vi "L2R_v2.vi"() -> ()   [LabVIEW 2022 SP3]
uses:
  <vilib>/regexp/Match Regular Expression.xnode
panel:
  in  "SET_term_z_offs":dbl=20.0 caption="terminal z \noffset:"
  in  "SET_term_moc":u16(ring) caption="terminal\nmovement:" items=["none", "inside", "-X", "-Y", "Z only"]
  in  "SET_x_offs":dbl caption="X offset:"
  in  "SET_y_offs":dbl caption="Y offset:"
  out "OUT_choice":bool
  out "OUT_file_num":i32 caption="split files created"
  out "CONV_splitting":bool caption="FILE SPLITTING"
  out "OUT_comm_lines":i32 caption="command lines found"
  in  "SET_max_lines":i32=2000 caption="max. file lines"
  in  "SET_tool_angl":bool caption="tool \nangulation:"
  out "FILE_name_old":string caption="old\nfilename:"
  in  "FILE_name_new":string caption="new \nfilename:"
  in  "SET_zone":i32=10 caption="zone:"
  in  "SET_tool":string="tool0" caption="tool:"
  in  "SET_movtype":u16(ring) caption="movement \ntype:" items=["LINEAR", "JOINT"]
  out "ERR_write_file":errorcluster
  out "OUT_rapid":string caption="RAPID string"
  out "CONV_running":bool caption="CONVERSION RUNNING"
  out "ERR_read_file":errorcluster caption="read file error"
  in  "FILE_path":path caption="file path:\n(dialog)"
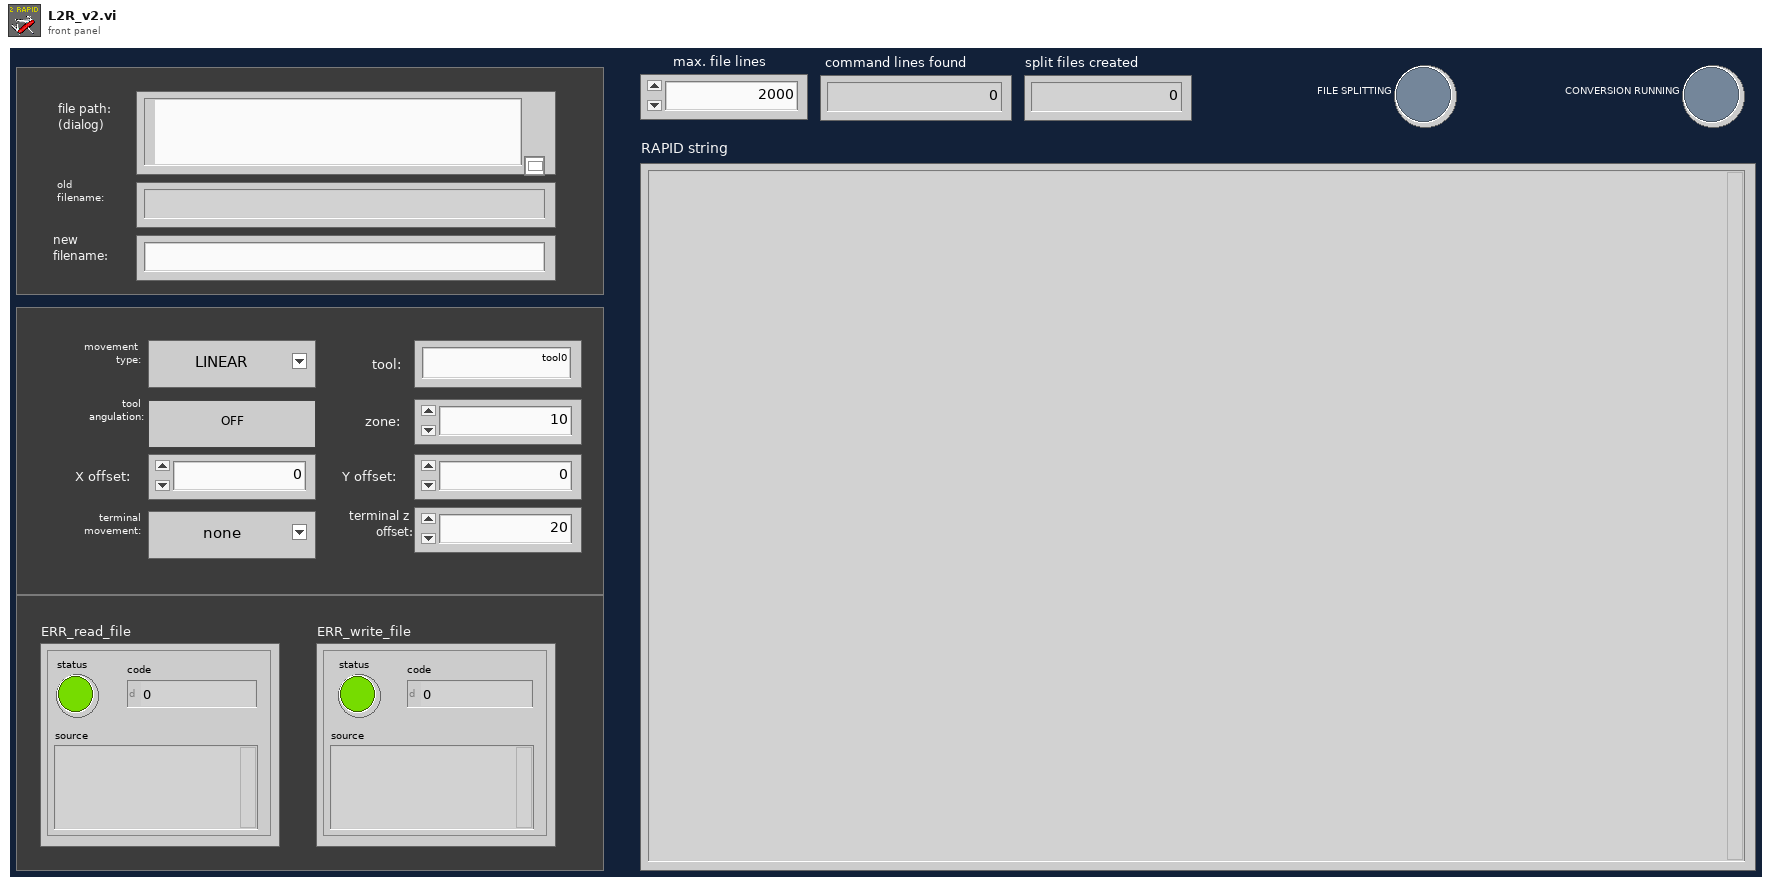
[diagram p1: front panel]
types:
  T1 = enum16{"open", "replace", "create", "open or create", "replace or create", "replace or create with confirmation"}
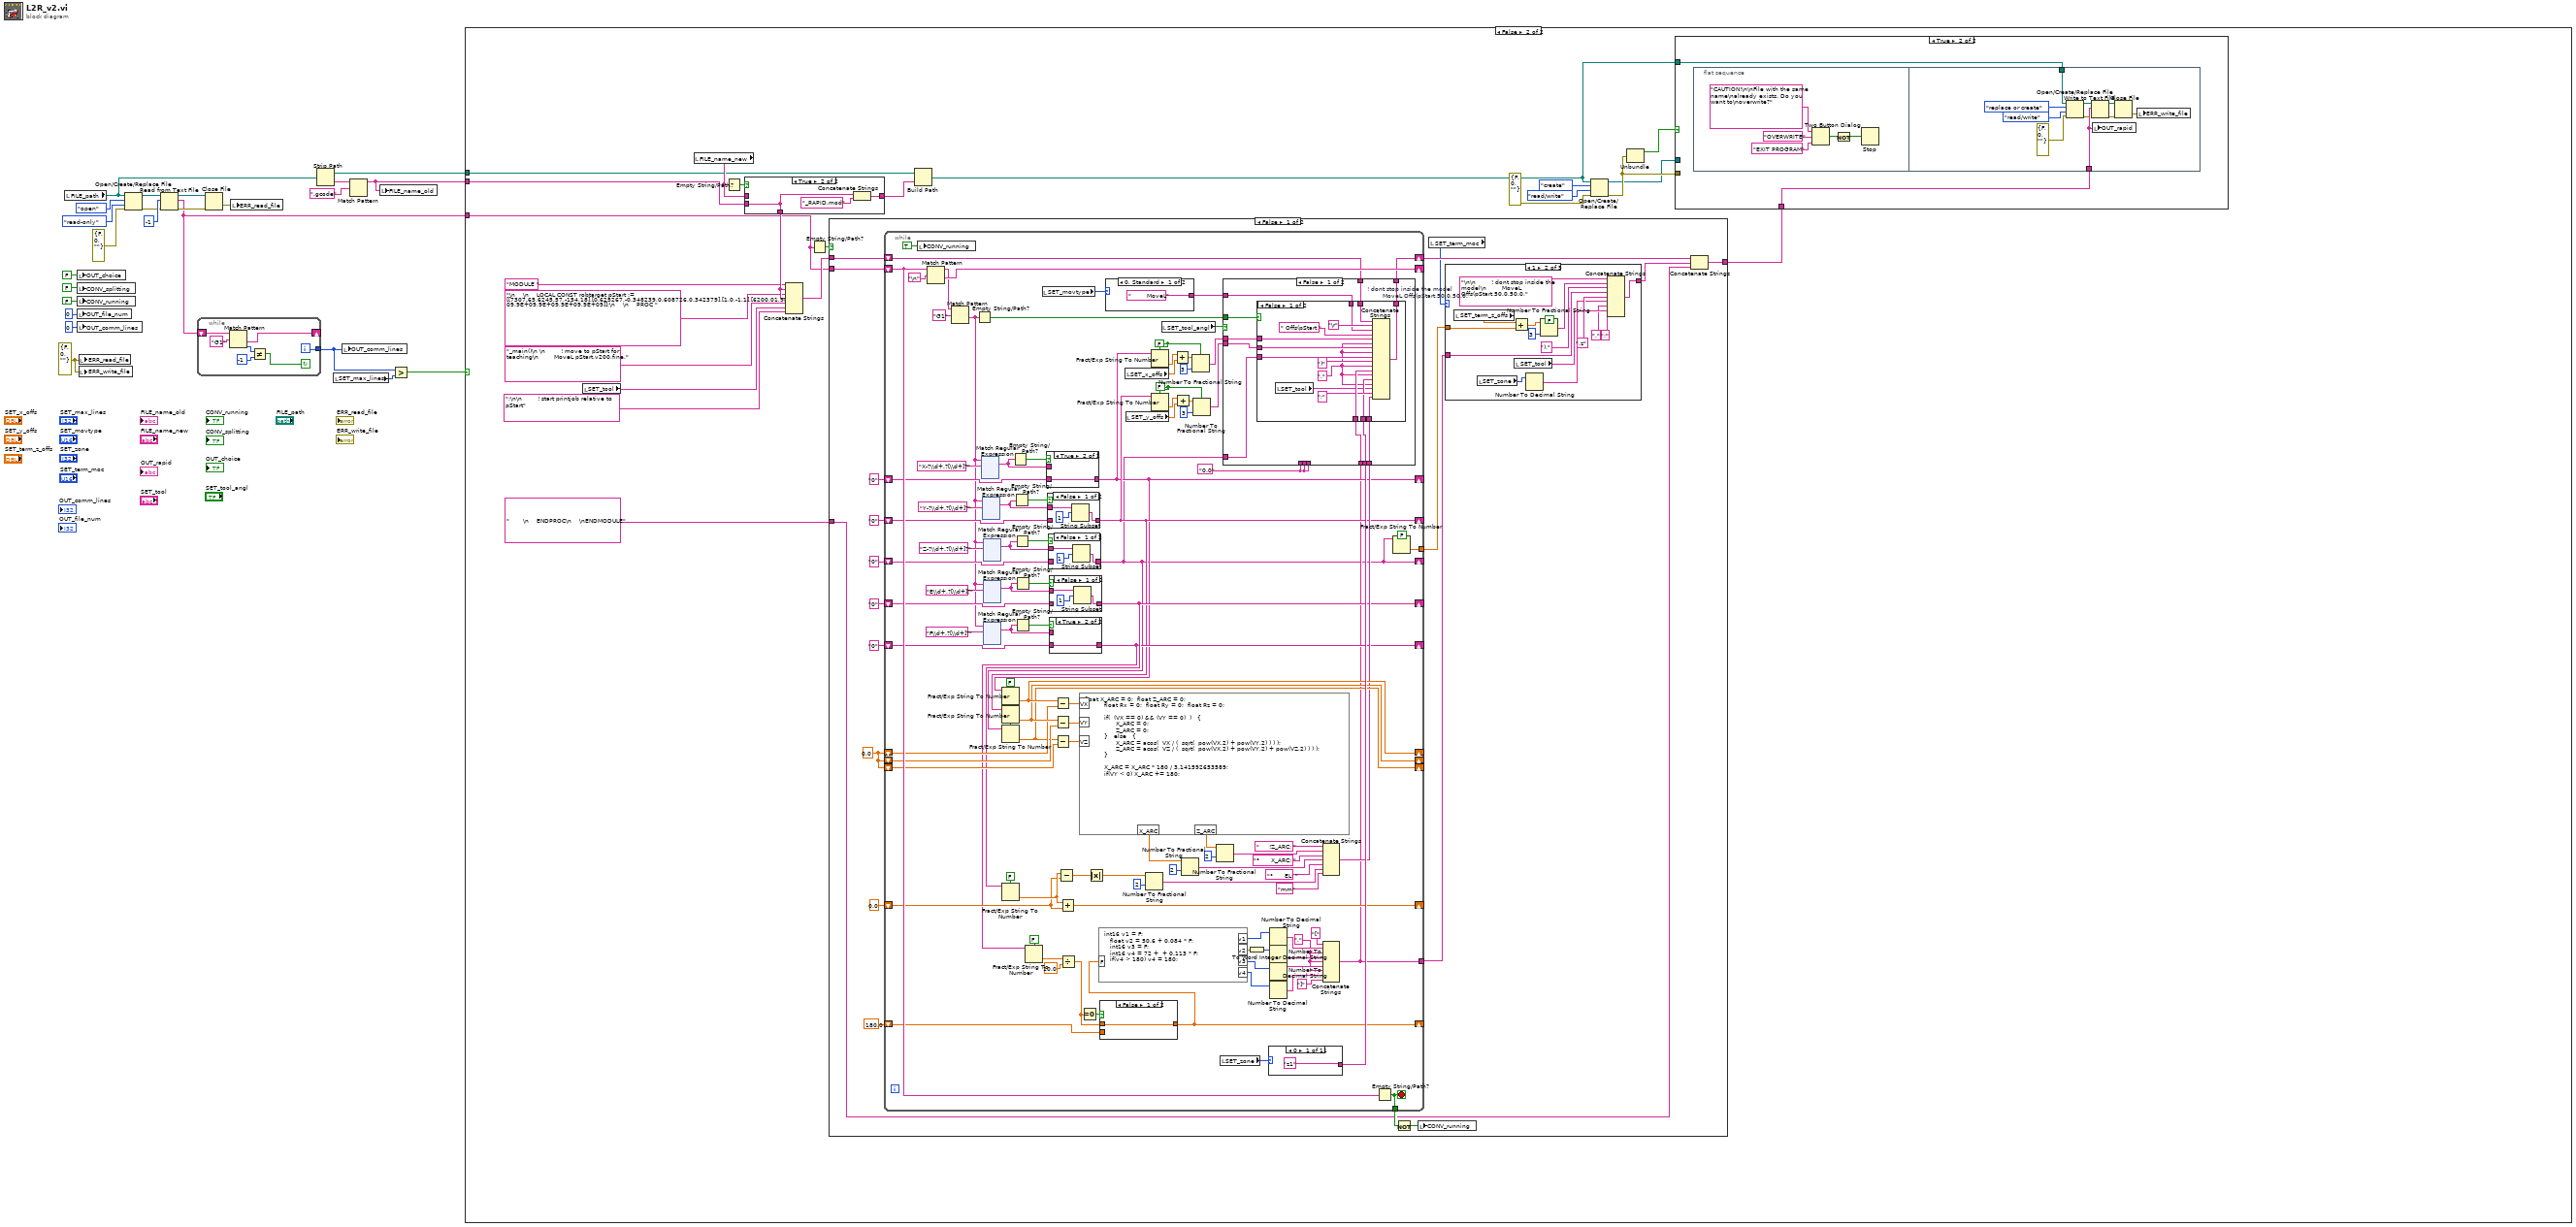
[diagram p0: block diagram]
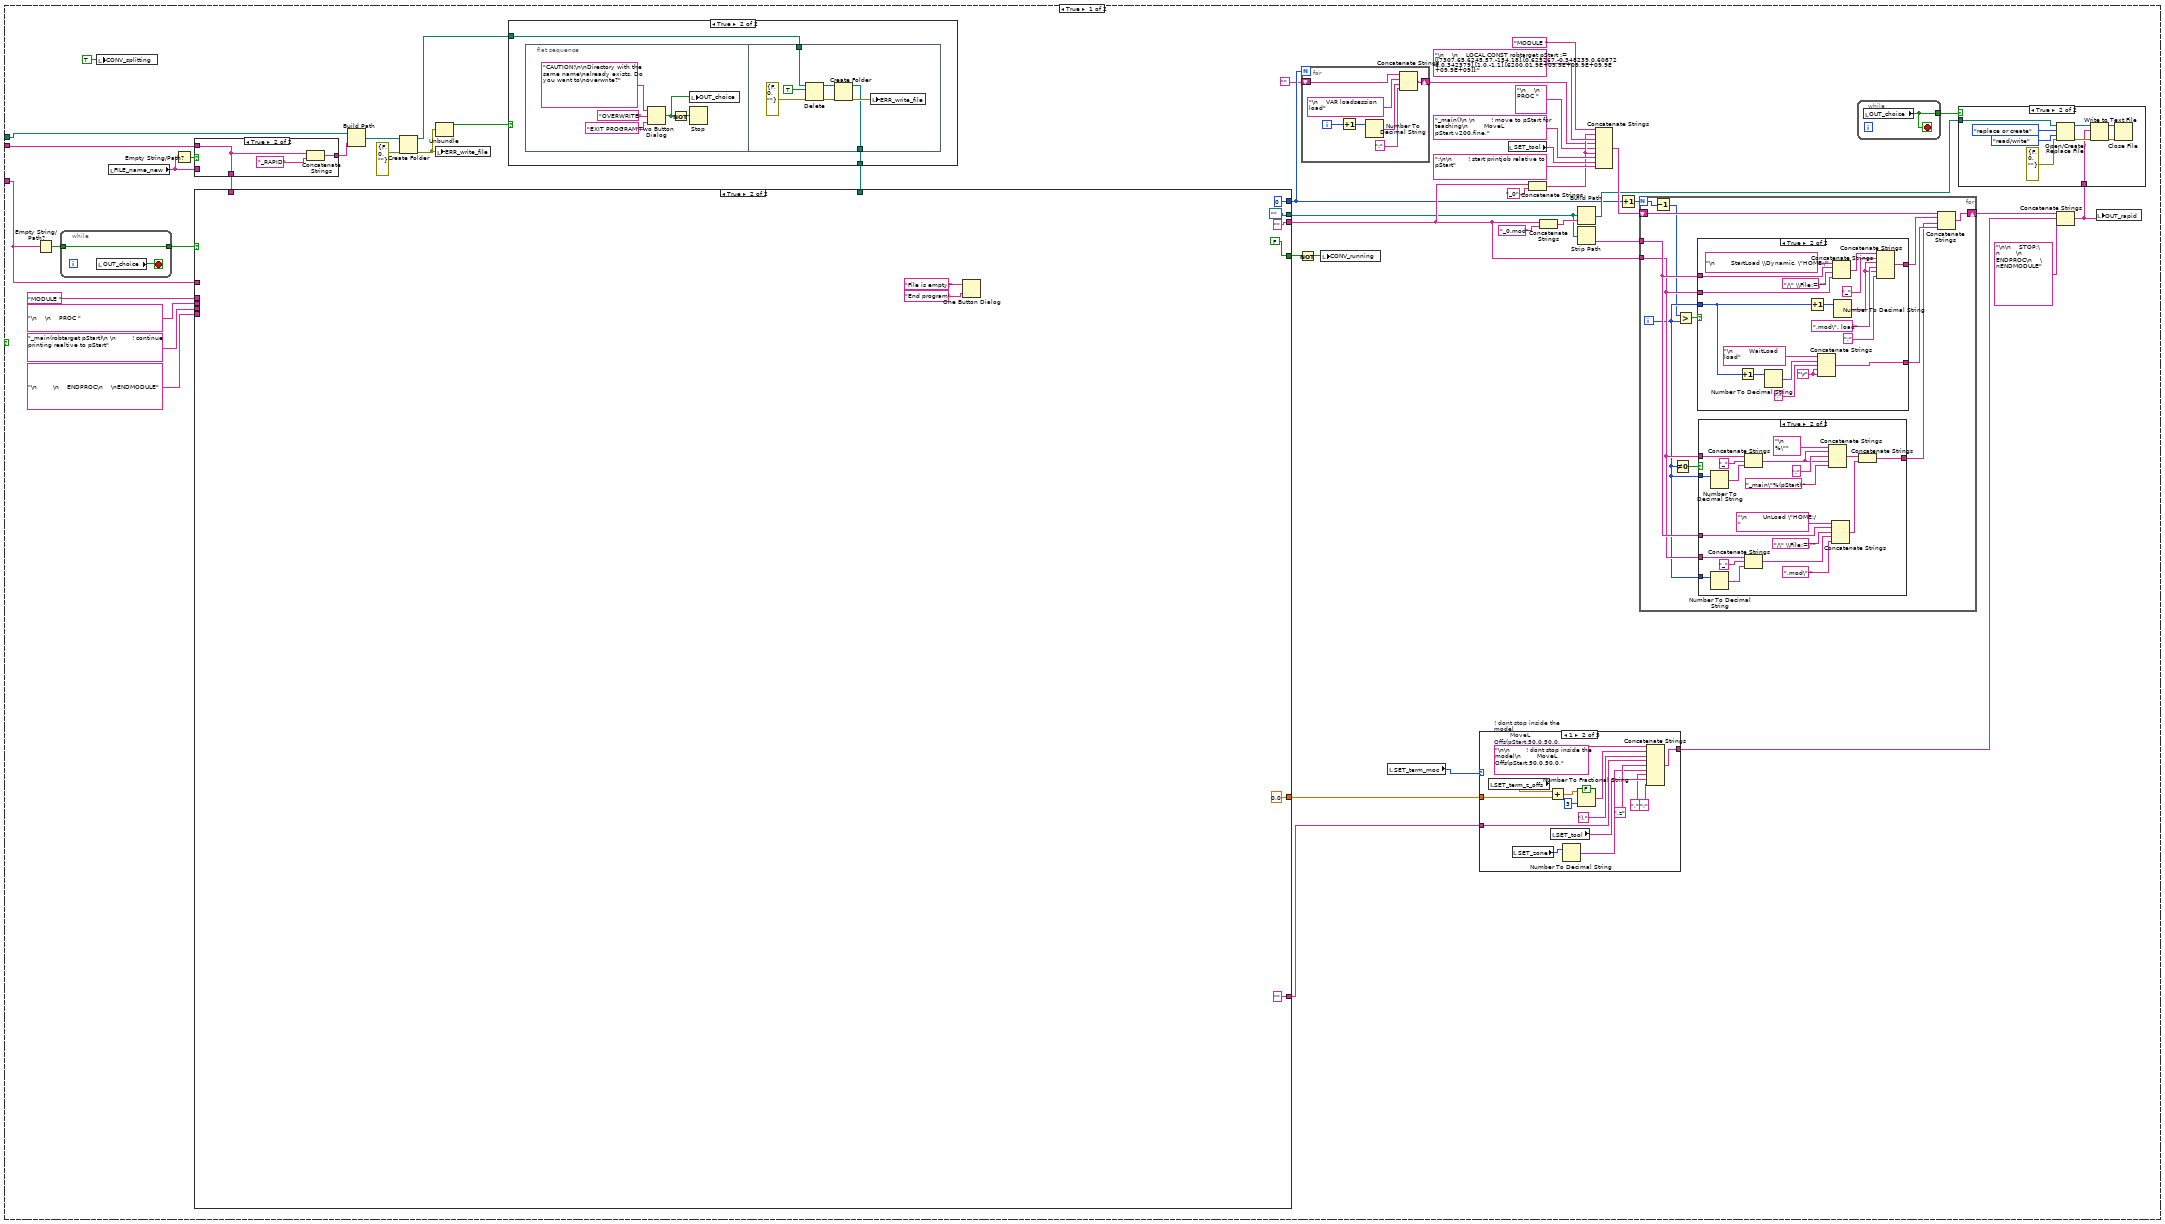
[diagram p2: hidden frame]
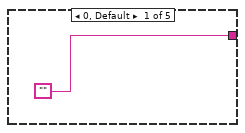
[diagram p3: hidden frame]
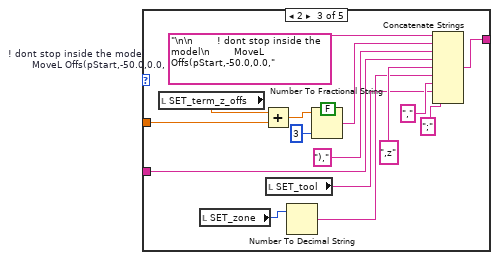
[diagram p4: hidden frame]
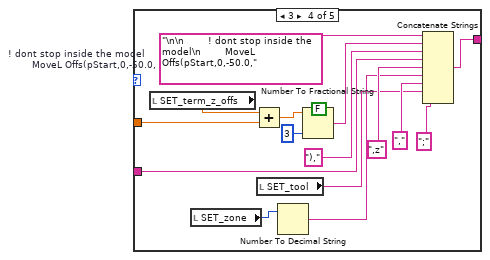
[diagram p5: hidden frame]
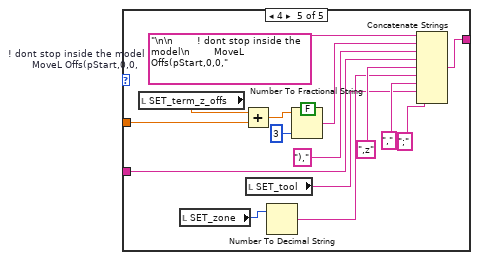
[diagram p6: hidden frame]
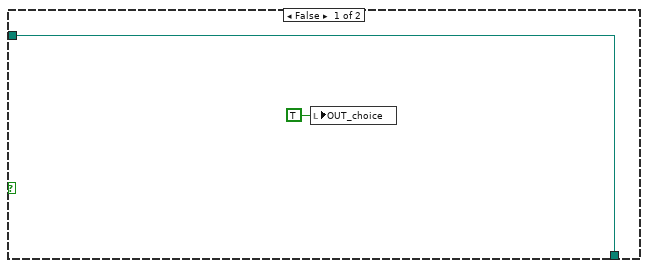
[diagram p8: hidden frame]
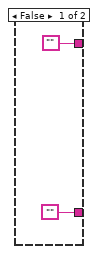
[diagram p9: hidden frame]
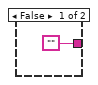
[diagram p10: hidden frame]
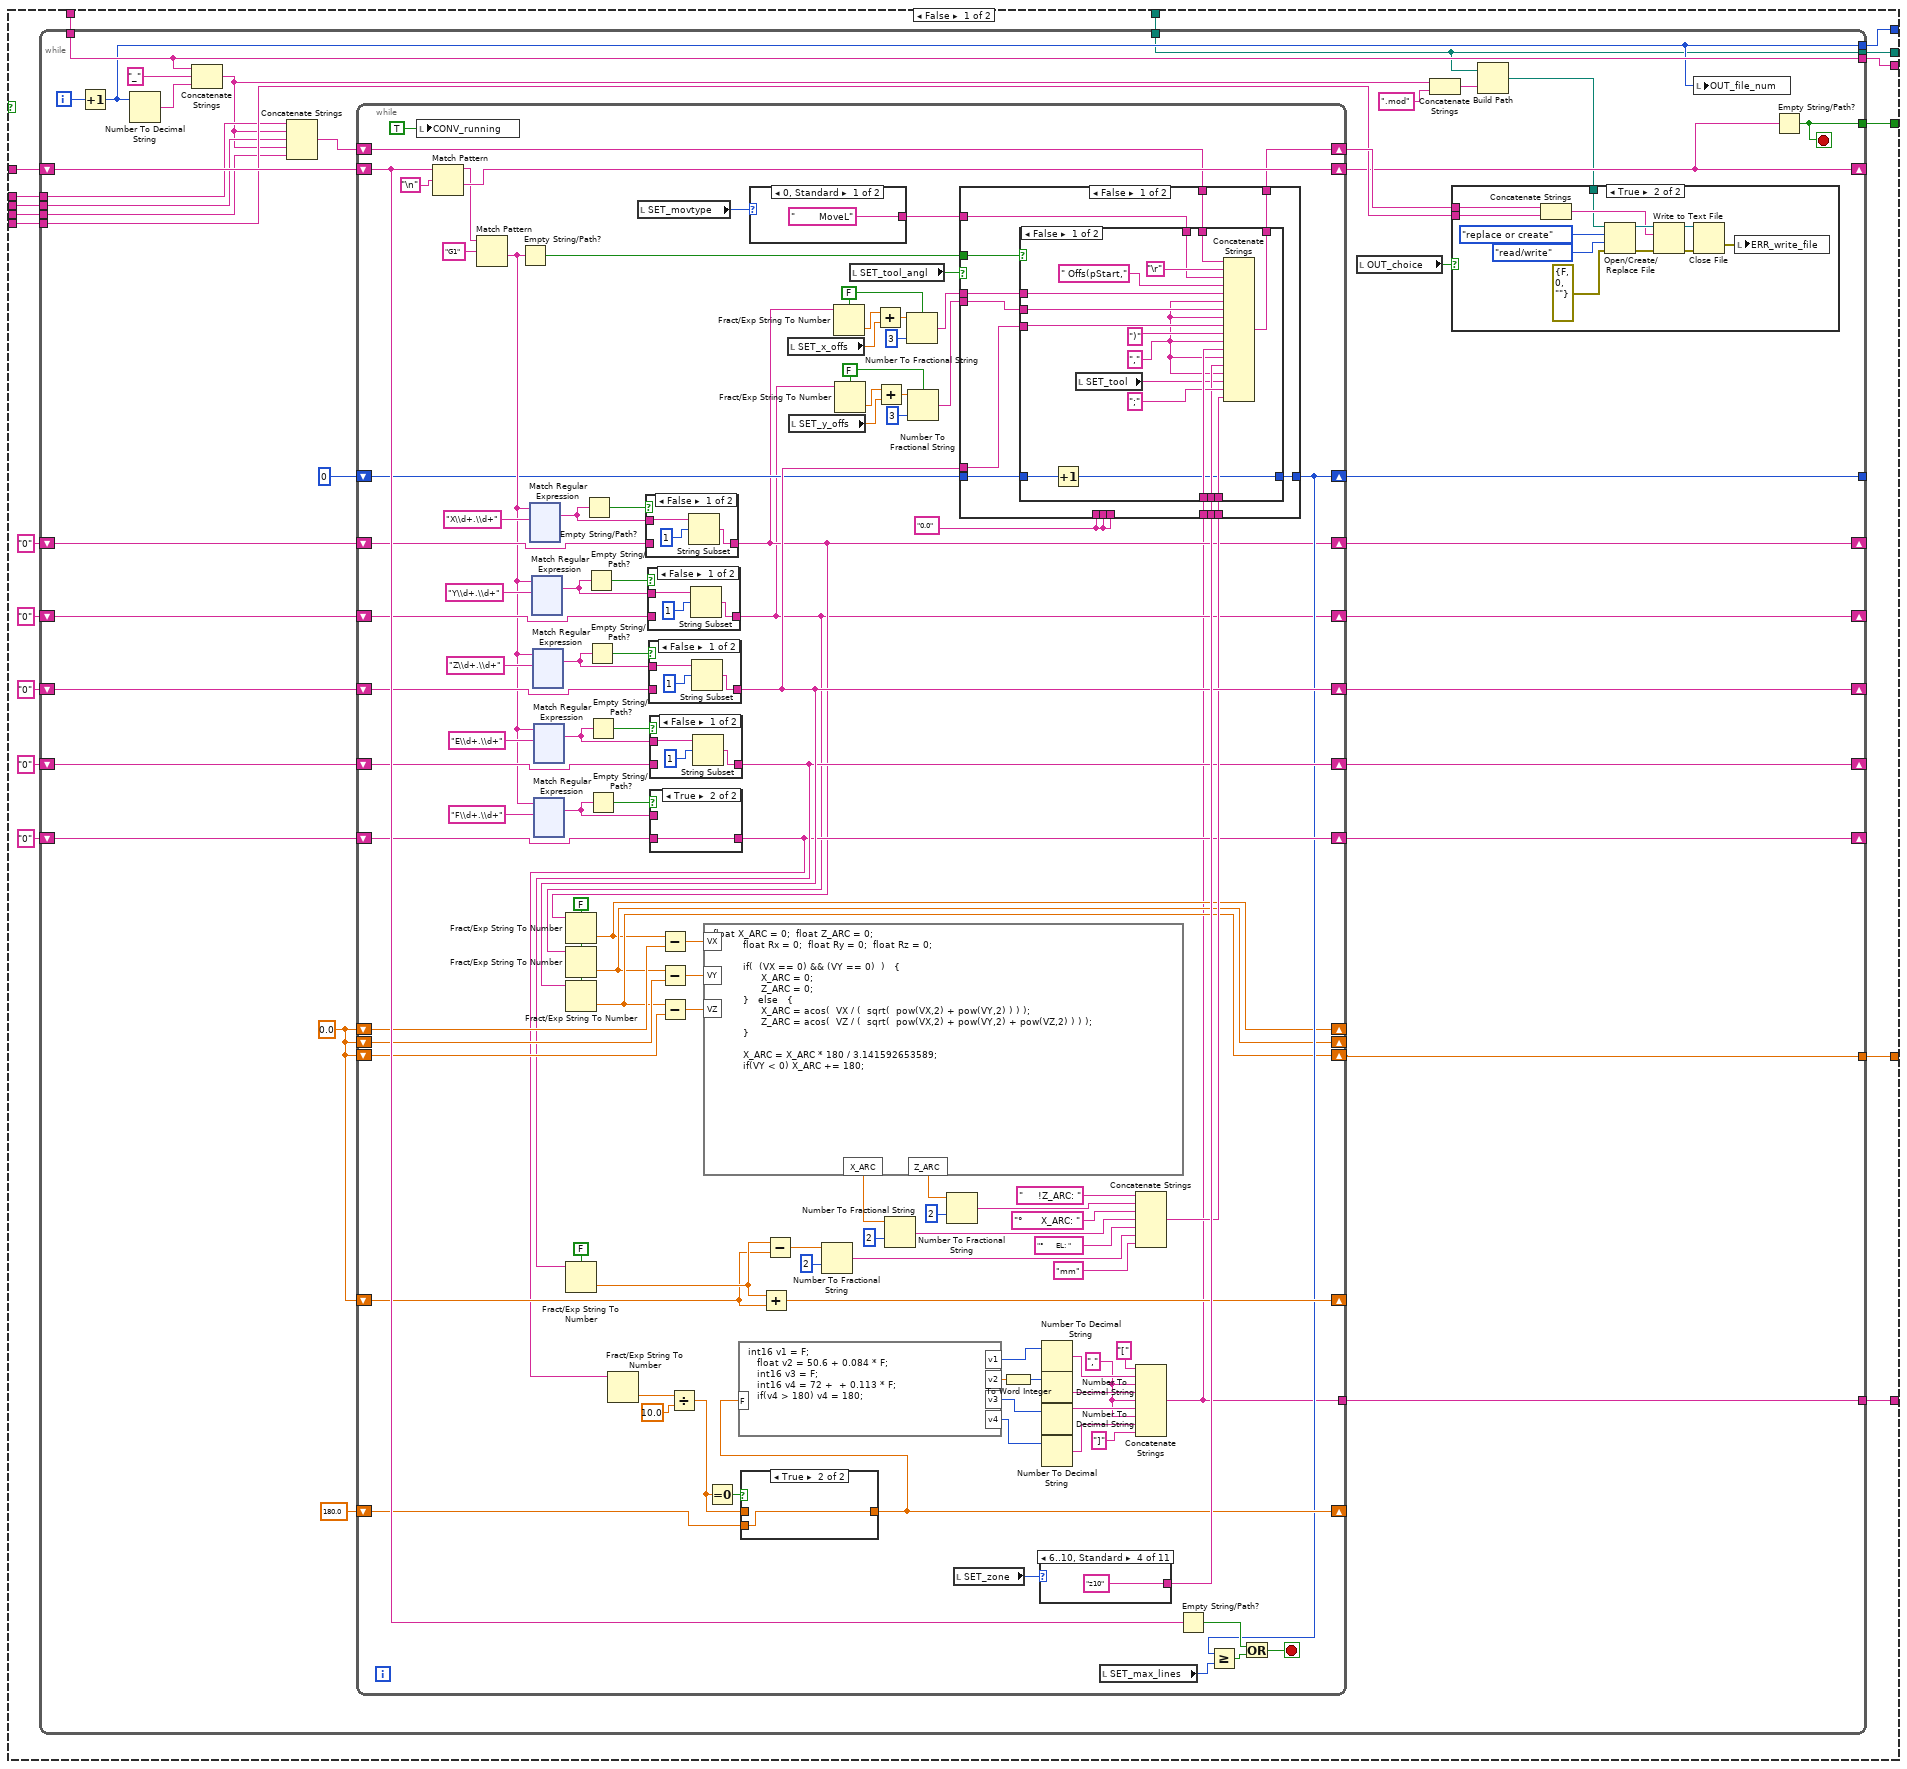
[diagram p12: hidden frame]
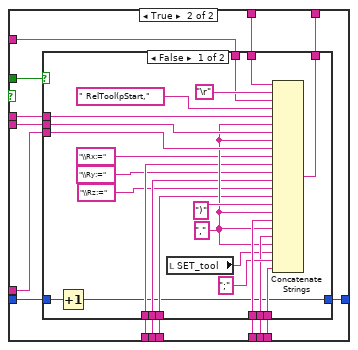
[diagram p16: hidden frame]
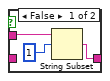
[diagram p18: hidden frame]
diagram:
  w5 = errorcluster {"status"=FALSE, "code"=0, "source"=""} ("ERR_write_file")
  n1 = local read "FILE_path"() -> (w9:path)
  n2 = local write "OUT_choice"(FALSE ("running")) -> ()
  n3 = local write "CONV_splitting"(FALSE ("running")) -> ()
  n4 = local write "CONV_running"(FALSE ("running")) -> ()
  n5 = local write "OUT_file_num"(0 ("OUT_file_num")) -> ()
  n6 = local write "OUT_comm_lines"(0 ("OUT_file_num")) -> ()
  n7 = local write "ERR_read_file"(w5) -> ()
  n8 = local write "ERR_write_file"(w5) -> ()
  n9 = Open/Create/Replace File(file path (use dialog)=w9, error in=errorcluster {"status"=FALSE, "code"=0, "source"=""}, operation (0:open)=T1."open", access (0:read/write)=enum16{"read/write", "read-only", "write-only"}."read-only") -> (refnum out=w20:refnum<file>, error out=w19:errorcluster)  [unwired: 2 in, 1 out]
  n10 = Read from Text File(file (use dialog)=w20, count=-1, error in=w19) -> (refnum out=w18:refnum<file>, text=w1:string, error out=w17:errorcluster)  [unwired: 1 in, 1 out]
  n11 = while {
    shift-right: [w29] -> _
    shift-left: w1 -> [w31]
    tunnel: [w25] -> w7
    i -> [w25]
    stop <- w26 continue-if-true
    n12 = Match Pattern(string=w31, regular expression="G1") -> (after substring=w29:string, offset past match=w28:i32)  [unwired: 1 in, 2 out]
    n13 = Not Equal?(x=w28, y=-1) -> (x != y?=w26:bool)
  }
  n14 = Close File(refnum=w18, error in=w17) -> (error out=w10:errorcluster)  [unwired: 1 out]
  n15 = local write "ERR_read_file"(w10) -> ()
  n16 = Strip Path(path=w9) -> (stripped path=w13:path, name=w15:string)
  n17 = local read "SET_max_lines"() -> (w11:i32)
  n18 = local write "OUT_comm_lines"(w7) -> ()
  n19 = Match Pattern(string=w15, regular expression=".gcode") -> (before substring=w8:string)  [unwired: 1 in, 3 out]
  n20 = local write "FILE_name_old"(w8) -> ()
  n21 = Greater?(x=w7, y=w11) -> (0:w12:bool)
  n22 = case shown="False" w12 {
    tunnel: w13 -> [w72 w1121]
    tunnel: w8 -> [w80 w1126]
    tunnel: w1 -> [w78 w1123]
    frame True {
      n23 = Empty String/Path?(string/path=w78) -> (empty?=w47:bool)
      n24 = while {
        tunnel: w47 -> [w154]
        tunnel: [w154] -> w46
        stop <- w155 stop-if-true
        n25 = local read "OUT_choice"() -> (w155:bool)
      }
      n26 = local write "CONV_splitting"(TRUE ("running")) -> ()
      n27 = local read "FILE_name_new"() -> (w77:string)
      n28 = Empty String/Path?(string/path=w77) -> (empty?=w79:bool)
      n29 = case shown="True" w79 {
        tunnel: w80 -> [_ w235]
        tunnel: w77 -> [w234 _]
        tunnel: [w234 w237] -> w70
        tunnel: [w234 w235] -> w74
        frame False {
        }
        frame True {
          n30 = Concatenate Strings(w235, "_RAPID" ("string")) -> (w237:string)
        }
      }
      n31 = Build Path(base path=w72, name or relative path=w70) -> (appended path=w71:path)
      n32 = Create Folder(path (use dialog)=w71, error in=errorcluster {"status"=FALSE, "code"=0, "source"=""}) -> (created path=w45:path, error out=w50:errorcluster)  [unwired: 1 in, 1 out]
      n33 = Unbundle(w50) -> ("status"=w49:bool)  [unwired: 2 out]
      n34 = local write "ERR_write_file"(w50) -> ()
      n35 = case shown="True" w49 {
        tunnel: w45 -> [w165 w168]
        tunnel: [w165 w167] -> w44
        frame False {
          n36 = local write "OUT_choice"(TRUE ("OUT_choice")) -> ()
        }
        frame True {
          n37 = flat-sequence {
            tunnel: w168 -> [w180]
            tunnel: [w174] -> w167
            frame #0 {
              n38 = Two Button Dialog(message="CAUTION!\n\nDirectory with the same name\nalready exists. Do you want to\noverwrite?", 1:"EXIT PROGRAM" ("F button name (\"Cancel\")"), 2:"OVERWRITE" ("T button name (\"OK\")")) -> (T button?=w169:bool)
              n39 = Not(x=w169) -> (.not. x?=w170:bool)
              n40 = Stop(stop? (T)=w170) -> ()
              n41 = local write "OUT_choice"(w169) -> ()
            }
            frame #1 {
              n42 = Delete(path (use dialog)=w180, entire hierarchy (F)=TRUE, error in=errorcluster {"status"=FALSE, "code"=0, "source"=""}) -> (deleted path=w178:path, error out=w177:errorcluster)  [unwired: 2 in, 1 out]
              n43 = Create Folder(path (use dialog)=w178, error in=w177) -> (created path=w174:path, error out=w175:errorcluster)  [unwired: 1 in, 1 out]
              n44 = local write "ERR_write_file"(w175) -> ()
            }
          }
        }
      }
      n45 = case shown="True" w46 {
        tunnel: w78 -> [w255 _]
        tunnel: "\n        \n    ENDPROC\n    \nENDMODULE" -> [w254 _]
        tunnel: [w253 FALSE] -> w75
        tunnel: w74 -> [w252 _]
        tunnel: "MODULE " -> [w251 _]
        tunnel: "\n    \n    PROC " -> [w250 _]
        tunnel: "_main(robtarget pStart)\n \n        ! continue printing realtive to pStart" -> [w249 _]
        tunnel: [w246 0 ("OUT_file_num")] -> w39
        tunnel: [w248 path "" ("created path")] -> w42
        tunnel: [w247 "" ("name")] -> w43
        tunnel: w44 -> [w245 _]
        tunnel: [w239 ""] -> w34
        tunnel: [w238 0.0] -> w35
        frame False {
          n46 = while {
            tunnel: w254 -> [w288]
            tunnel: [w287] -> w253
            tunnel: w252 -> [w274]
            tunnel: w251 -> [w286]
            tunnel: w250 -> [w285]
            tunnel: w249 -> [w284]
            shift-right: [w279] -> _
            shift-left: w255 -> [w291]
            tunnel: [w271] -> w248
            tunnel: [w274] -> w247
            tunnel: [w272] -> w246
            tunnel: w245 -> [w271]
            shift-right: [w264] -> _
            shift-left: "0" ("whole match") -> [w270]
            shift-right: [w263] -> _
            shift-left: "0" ("whole match") -> [w269]
            shift-right: [w262] -> _
            shift-left: "0" ("whole match") -> [w268]
            shift-right: [w261] -> _
            shift-left: "0" ("whole match") -> [w267]
            shift-right: [w260] -> _
            shift-left: "0" ("whole match") -> [w266]
            tunnel: [w265] -> _
            tunnel: [w257] -> w239
            tunnel: [w256] -> w238
            i -> [w282]
            stop <- w287 stop-if-true
            w258 = 0.0
            n47 = Increment(x=w282) -> (x+1=w272:i32)
            n48 = Number To Decimal String(number=w272) -> (decimal integer string=w280:string)  [unwired: 1 in]
            n49 = Concatenate Strings(w274, "_" ("string"), w280) -> (w277:string)
            n50 = Concatenate Strings(w286, w277, w285, w277, w284) -> (w283:string)
            n51 = while {
              shift-right: [w407] -> w279
              shift-left: w291 -> [w409]
              shift-right: [w403] -> w290
              shift-left: w283 -> [w404]
              shift-right: [w305] -> _
              shift-left: w258 -> [w386]
              shift-right: [w306] -> _
              shift-left: w258 -> [w385]
              shift-right: [w307] -> w256
              shift-left: w258 -> [w352]
              shift-right: [w321] -> w264
              shift-left: w270 -> [w378]
              shift-right: [w309] -> w263
              shift-left: w269 -> [w365]
              shift-right: [w361] -> w262
              shift-left: w268 -> [w364]
              shift-right: [w344] -> w261
              shift-left: w267 -> [w363]
              shift-right: [w335] -> w260
              shift-left: w266 -> [w362]
              shift-right: [w339] -> _
              shift-left: w258 -> [w337]
              shift-right: [w331] -> _
              shift-left: 180.0 -> [w332]
              shift-right: [w322] -> w265
              shift-left: 0 -> [w323]
              tunnel: [w304] -> w257
              stop <- w326 stop-if-true
              w313 = FALSE ("Systemdezimalzeichen verwenden (T)")
              w317 = FALSE ("Systemdezimalzeichen verwenden (T)")
              w336 = "0.0"
              w357 = FALSE ("use system decimal point (T)")
              w389 = ","
              n52 = local write "CONV_running"(TRUE ("running")) -> ()
              n53 = Match Pattern(string=w409, regular expression="\n") -> (before substring=w406:string, after substring=w407:string)  [unwired: 1 in, 2 out]
              n54 = Match Pattern(string=w406, regular expression="G1") -> (after substring=w360:string)  [unwired: 1 in, 3 out]
              n55 = Empty String/Path?(string/path=w360) -> (empty?=w402:bool)
              n56 = xnode "Match Regular Expression"("input string"=w360, "regular expression"="X\\d+.\\d+") -> ("whole match"=w379:string)  [unwired: 4 in, 4 out]
              n57 = xnode "Match Regular Expression"("input string"=w360, "regular expression"="Y\\d+.\\d+") -> ("whole match"=w377:string)  [unwired: 4 in, 4 out]
              n58 = xnode "Match Regular Expression"("input string"=w360, "regular expression"="Z\\d+.\\d+") -> ("whole match"=w372:string)  [unwired: 4 in, 4 out]
              n59 = xnode "Match Regular Expression"("input string"=w360, "regular expression"="E\\d+.\\d+") -> ("whole match"=w371:string)  [unwired: 4 in, 4 out]
              n60 = xnode "Match Regular Expression"("input string"=w360, "regular expression"="F\\d+.\\d+") -> ("whole match"=w366:string)  [unwired: 4 in, 4 out]
              n61 = Empty String/Path?(string/path=w379) -> (empty?=w380:bool)
              n62 = Empty String/Path?(string/path=w377) -> (empty?=w376:bool)
              n63 = Empty String/Path?(string/path=w372) -> (empty?=w373:bool)
              n64 = Empty String/Path?(string/path=w371) -> (empty?=w370:bool)
              n65 = Empty String/Path?(string/path=w366) -> (empty?=w367:bool)
              n66 = local read "SET_movtype"() -> (w330:u16)
              n67 = case shown="False" w380 {
                tunnel: w379 -> [w969 _]
                tunnel: [w967 w970] -> w321
                tunnel: w378 -> [_ w970]
                frame False {
                  n68 = String Subset(string=w969, offset (0)=1) -> (substring=w967:string)  [unwired: 1 in]
                }
                frame True {
                }
              }
              n69 = Fract/Exp String To Number(use system decimal point (T)=w357, string=w321) -> (number=w305:dbl)  [unwired: 2 in, 1 out]
              n70 = case shown="False" w376 {
                tunnel: w377 -> [w848 _]
                tunnel: [w846 w849] -> w309
                tunnel: w365 -> [_ w849]
                frame False {
                  n71 = String Subset(string=w848, offset (0)=1) -> (substring=w846:string)  [unwired: 1 in]
                }
                frame True {
                }
              }
              n72 = Fract/Exp String To Number(use system decimal point (T)=w357, string=w309) -> (number=w306:dbl)  [unwired: 2 in, 1 out]
              n73 = case shown="False" w373 {
                tunnel: w372 -> [w727 _]
                tunnel: [w725 w728] -> w361
                tunnel: w364 -> [_ w728]
                frame False {
                  n74 = String Subset(string=w727, offset (0)=1) -> (substring=w725:string)  [unwired: 1 in]
                }
                frame True {
                }
              }
              n75 = Fract/Exp String To Number(use system decimal point (T)=w357, string=w361) -> (number=w307:dbl)  [unwired: 2 in, 1 out]
              n76 = case shown="False" w370 {
                tunnel: w371 -> [w606 _]
                tunnel: [w604 w607] -> w344
                tunnel: w363 -> [_ w607]
                frame False {
                  n77 = String Subset(string=w606, offset (0)=1) -> (substring=w604:string)  [unwired: 1 in]
                }
                frame True {
                }
              }
              n78 = Fract/Exp String To Number(use system decimal point (T)=FALSE, string=w344) -> (number=w338:dbl)  [unwired: 2 in, 1 out]
              n79 = case shown="True" w367 {
                tunnel: w366 -> [w485 _]
                tunnel: [w483 w486] -> w335
                tunnel: w362 -> [_ w486]
                frame False {
                  n80 = String Subset(string=w485, offset (0)=1) -> (substring=w483:string)  [unwired: 1 in]
                }
                frame True {
                }
              }
              n81 = Fract/Exp String To Number(string=w335) -> (number=w359:dbl)  [unwired: 3 in, 1 out]
              n82 = Subtract(x=w305, y=w386) -> (x-y=w383:dbl)
              n83 = Subtract(x=w306, y=w385) -> (x-y=w384:dbl)
              n84 = Subtract(x=w307, y=w352) -> (x-y=w353:dbl)
              n85 = Divide(x=w359, y=10.0) -> (x/y=w333:dbl)
              n86 = formula code="float X_ARC = 0;  float Z_ARC = 0;\n          float Rx = 0;  float Ry = 0;  float Rz = 0;\n        \n          if(  (VX == 0) && (VY == 0)  )   {\n                X_ARC = 0;\n                Z_ARC = 0;\n          }   else   {\n                X_ARC = acos(  VX / (  sqrt(  pow(VX,2) + pow(VY,2) ) ) );\n                Z_ARC = acos(  VZ / (  sqrt(  pow(VX,2) + pow(VY,2) + pow(VZ,2) ) ) );\n          }\n        \n          X_ARC = X_ARC * 180 / 3.141592653589;\n          if(VY < 0) X_ARC += 180;"("VX"=w383, "VY"=w384, "VZ"=w353) -> ("X_ARC"=w351:dbl, "Z_ARC"=w349:dbl)
              n87 = Equal To 0?(x=w333) -> (x = 0?=w334:bool)
              n88 = case shown="True" w334 {
                tunnel: w333 -> [w410 _]
                tunnel: [w410 w411] -> w331
                tunnel: w332 -> [_ w411]
                frame False {
                }
                frame True {
                }
              }
              n89 = formula code="int16 v1 = F;\n   float v2 = 50.6 + 0.084 * F;\n   int16 v3 = F;\n   int16 v4 = 72 +  + 0.113 * F;\n   if(v4 > 180) v4 = 180;"("F"=w331) -> ("v1"=w398:i16, "v2"=w397:dbl, "v3"=w395:i16, "v4"=w394:i16)
              n90 = case shown="0, Standard" w330 {
                tunnel: ["        MoveL" "        MoveJ"] -> w401
                frame 0, Default {
                }
                frame 1 {
                }
              }
              n91 = Add(x=w338, y=w337) -> (x+y=w339:dbl)
              n92 = Subtract(x=w338, y=w337) -> (x-y=w340:dbl)
              n93 = local read "SET_x_offs"() -> (w316:dbl)
              n94 = local read "SET_y_offs"() -> (w314:dbl)
              n95 = Number To Fractional String(number=w340, precision (6)=i16 2) -> (F-format string=w341:string)  [unwired: 2 in]
              n96 = Fract/Exp String To Number(use system decimal point (T)=w317, string=w321) -> (number=w320:dbl)  [unwired: 2 in, 1 out]
              n97 = Fract/Exp String To Number(use system decimal point (T)=w313, string=w309) -> (number=w310:dbl)  [unwired: 2 in, 1 out]
              n98 = local read "SET_tool_angl"() -> (w328:bool)
              n99 = Add(x=w320, y=w316) -> (x+y=w319:dbl)
              n100 = Add(x=w310, y=w314) -> (x+y=w311:dbl)
              n101 = Number To Fractional String(number=w351, precision (6)=i16 2) -> (F-format string=w347:string)  [unwired: 2 in]
              n102 = Number To Fractional String(use system decimal point (T)=w317, number=w319, precision (6)=i16 3 ("Genauigkeit (6)")) -> (F-format string=w315:string)  [unwired: 1 in]
              n103 = Number To Fractional String(use system decimal point (T)=w313, number=w311, precision (6)=i16 3 ("Genauigkeit (6)")) -> (F-format string=w308:string)  [unwired: 1 in]
              n104 = Number To Fractional String(number=w349, precision (6)=i16 2) -> (F-format string=w348:string)  [unwired: 2 in]
              n105 = local read "SET_zone"() -> (w327:i32)
              n106 = To Word Integer(number=w397) -> (16bit integer=w396:i16)
              n107 = case shown="6..10, Standard" w327 {
                tunnel: ["z1" "z2" "z5" "z10" "z20" "z50" "z100" "z200" "z300" "z400" "z500"] -> w400
                frame 0 {
                }
                frame 1, 2 {
                }
                frame 3..5 {
                }
                frame 6..10, Default {
                }
                frame 11..20 {
                }
                frame 21..50 {
                }
                frame 51..100 {
                }
                frame 101..200 {
                }
                frame 201..300 {
                }
                frame 301..400 {
                }
                frame 401..500 {
                }
              }
              n108 = Number To Decimal String(number=w398) -> (decimal integer string=w392:string)  [unwired: 1 in]
              n109 = Number To Decimal String(number=w396) -> (decimal integer string=w391:string)  [unwired: 1 in]
              n110 = Number To Decimal String(number=w395) -> (decimal integer string=w390:string)  [unwired: 1 in]
              n111 = Number To Decimal String(number=w394) -> (decimal integer string=w388:string)  [unwired: 1 in]
              n112 = local read "SET_max_lines"() -> (w324:i32)
              n113 = Concatenate Strings("     !Z_ARC: ", w348, "°      X_ARC: ", w347, "°      EL: " ("string"), w341, "mm" ("string")) -> (w345:string)
              n114 = Concatenate Strings("[", w392, w389, w391, w389, w390, w389, w388, "]") -> (w304:string)
              n115 = case shown="False" w328 {
                tunnel: w404 -> [w423 w457]
                tunnel: [w422 w456] -> w403
                tunnel: w402 -> [w421 w455]
                tunnel: w401 -> [w420 w454]
                tunnel: w400 -> [w419 w453]
                tunnel: w304 -> [w418 w452]
                tunnel: w308 -> [w417 w451]
                tunnel: w315 -> [w416 w450]
                tunnel: w361 -> [w415 w449]
                tunnel: w345 -> [w414 w448]
                tunnel: w336 -> [_ w447]
                tunnel: w336 -> [_ w446]
                tunnel: w336 -> [_ w445]
                tunnel: [w412 w444] -> w322
                tunnel: w323 -> [w413 w443]
                frame False {
                  n116 = case shown="False" w421 {
                    tunnel: w423 -> [w440 w442]
                    tunnel: w416 -> [w437 _]
                    tunnel: w417 -> [w436 _]
                    tunnel: w415 -> [w435 _]
                    tunnel: w418 -> [w434 _]
                    tunnel: [w433 w442] -> w422
                    tunnel: w420 -> [w431 _]
                    tunnel: w419 -> [w429 _]
                    tunnel: w414 -> [w426 _]
                    tunnel: w413 -> [w425 w441]
                    tunnel: [w424 w441] -> w412
                    frame False {
                      w428 = ","
                      n117 = Increment(x=w425) -> (x+1=w424:i32)
                      n118 = local read "SET_tool"() -> (w427:string)
                      n119 = Concatenate Strings(w440, "\r", w431, " Offs(pStart,", w437, w428, w436, w428, w435, ")" ("string"), w428, w434, w428, w429, w428, w427, ";" ("string"), w426) -> (w433:string)
                    }
                    frame True {
                    }
                  }
                }
                frame True {
                  n120 = case shown="False" w455 {
                    tunnel: w457 -> [w480 w482]
                    tunnel: w450 -> [w477 _]
                    tunnel: w451 -> [w476 _]
                    tunnel: w449 -> [w475 _]
                    tunnel: w452 -> [w474 _]
                    tunnel: [w473 w482] -> w456
                    tunnel: w454 -> [w471 _]
                    tunnel: w453 -> [w469 _]
                    tunnel: w448 -> [w466 _]
                    tunnel: w447 -> [w465 _]
                    tunnel: w446 -> [w464 _]
                    tunnel: w445 -> [w463 _]
                    tunnel: [w459 w481] -> w444
                    tunnel: w443 -> [w458 w481]
                    frame False {
                      w468 = ","
                      n121 = Increment(x=w458) -> (x+1=w459:i32)
                      n122 = local read "SET_tool"() -> (w467:string)
                      n123 = Concatenate Strings(w480, "\r", w471, " RelTool(pStart,", w477, w468, w476, w468, w475, "\\Rx:=" ("string"), w465, "\\Ry:=" ("string"), w464, "\\Rz:=" ("string"), w463, ")" ("string"), w468, w474, w468, w469, w468, w467, ";" ("string"), w466) -> (w473:string)
                    }
                    frame True {
                    }
                  }
                }
              }
              n124 = Empty String/Path?(string/path=w409) -> (empty?=w399:bool)
              n125 = Greater Or Equal?(x=w322, y=w324) -> (x >= y?=w325:bool)
              n126 = Or(x=w399, y=w325) -> (x .or. y?=w326:bool)
            }
            n127 = local read "OUT_choice"() -> (w273:bool)
            n128 = Concatenate Strings(w277, ".mod") -> (w276:string)
            n129 = Build Path(base path=w271, name or relative path=w276) -> (appended path=w275:path)
            n130 = case shown="True" w273 {
              tunnel: w290 -> [_ w303]
              tunnel: w288 -> [_ w302]
              tunnel: w275 -> [_ w292]
              frame False {
              }
              frame True {
                n131 = Concatenate Strings(w303, w302) -> (w293:string)
                n132 = Open/Create/Replace File(file path (use dialog)=w292, error in=errorcluster {"status"=FALSE, "code"=0, "source"=""}, operation (0:open)=T1."replace or create", access (0:read/write)=enum16{"read/write", "read-only", "write-only"}."read/write") -> (refnum out=w297:refnum<file>, error out=w298:errorcluster)  [unwired: 2 in, 1 out]
                n133 = Write to Text File(file (use dialog)=w297, text=w293, error in=w298) -> (refnum out=w299:refnum<file>, error out=w300:errorcluster)  [unwired: 1 in, 1 out]
                n134 = Close File(refnum=w299, error in=w300) -> (error out=w301:errorcluster)  [unwired: 1 out]
                n135 = local write "ERR_write_file"(w301) -> ()
              }
            }
            n136 = local write "OUT_file_num"(w272) -> ()
            n137 = Empty String/Path?(string/path=w279) -> (empty?=w287:bool)
          }
        }
        frame True {
          n138 = One Button Dialog(message="File is empty!", button name ("OK")="End program") -> ()  [unwired: 1 out]
        }
      }
      n139 = Not(x=w75) -> (.not. x?=w76:bool)
      n140 = for {
        N: w39 -> [_]
        shift-right: [w147] -> w37
        shift-left: "" -> [w146]
        i -> [w151]
        n141 = Increment(x=w151) -> (x+1=w152:i32)
        n142 = Number To Decimal String(number=w152) -> (decimal integer string=w149:string)  [unwired: 1 in]
        n143 = Concatenate Strings(w146, "\n    VAR loadsession load", w149, ";" ("string")) -> (w147:string)
      }
      n144 = local write "CONV_running"(w76) -> ()
      n145 = local read "SET_term_moc"() -> (w32:u16)
      n146 = case shown="1" w32 {
        tunnel: ["" w97 w113 w129 w145] -> w33
        tunnel: w34 -> [_ w94 w110 w126 w142]
        tunnel: w35 -> [_ w92 w108 w124 w140]
        frame 0, Default {
        }
        frame 1 {
          w96 = "\n\n        ! dont stop inside the model\n        MoveL Offs(pStart,50.0,50.0,"  # ! dont stop inside the model         MoveL Offs(pStart,50.0,50.0,
          n147 = local read "SET_term_z_offs"() -> (w88:dbl)
          n148 = local read "SET_zone"() -> (w85:i32)
          n149 = Add(x=w88, y=w92) -> (x+y=w89:dbl)
          n150 = local read "SET_tool"() -> (w83:string)
          n151 = Number To Decimal String(number=w85) -> (decimal integer string=w84:string)  [unwired: 1 in]
          n152 = Number To Fractional String(use system decimal point (T)=FALSE ("Systemdezimalzeichen verwenden (T)"), number=w89, precision (6)=i16 3 ("Genauigkeit (6)")) -> (F-format string=w90:string)  [unwired: 1 in]
          n153 = Concatenate Strings(w96, w90, "),", w94, ",z", w84, "," ("String"), w83, ";" ("String")) -> (w97:string)
        }
        frame 2 {
          w112 = "\n\n        ! dont stop inside the model\n        MoveL Offs(pStart,-50.0,0.0,"  # ! dont stop inside the model         MoveL Offs(pStart,-50.0,0.0,
          n154 = local read "SET_term_z_offs"() -> (w104:dbl)
          n155 = local read "SET_zone"() -> (w101:i32)
          n156 = Add(x=w104, y=w108) -> (x+y=w105:dbl)
          n157 = local read "SET_tool"() -> (w98:string)
          n158 = Number To Decimal String(number=w101) -> (decimal integer string=w99:string)  [unwired: 1 in]
          n159 = Number To Fractional String(use system decimal point (T)=FALSE ("Systemdezimalzeichen verwenden (T)"), number=w105, precision (6)=i16 3 ("Genauigkeit (6)")) -> (F-format string=w106:string)  [unwired: 1 in]
          n160 = Concatenate Strings(w112, w106, "),", w110, ",z", w99, "," ("String"), w98, ";" ("String")) -> (w113:string)
        }
        frame 3 {
          w128 = "\n\n        ! dont stop inside the model\n        MoveL Offs(pStart,0,-50.0,"  # ! dont stop inside the model         MoveL Offs(pStart,0,-50.0,
          n161 = local read "SET_term_z_offs"() -> (w120:dbl)
          n162 = local read "SET_zone"() -> (w117:i32)
          n163 = Add(x=w120, y=w124) -> (x+y=w121:dbl)
          n164 = local read "SET_tool"() -> (w114:string)
          n165 = Number To Decimal String(number=w117) -> (decimal integer string=w115:string)  [unwired: 1 in]
          n166 = Number To Fractional String(use system decimal point (T)=FALSE ("Systemdezimalzeichen verwenden (T)"), number=w121, precision (6)=i16 3 ("Genauigkeit (6)")) -> (F-format string=w122:string)  [unwired: 1 in]
          n167 = Concatenate Strings(w128, w122, "),", w126, ",z", w115, "," ("String"), w114, ";" ("String")) -> (w129:string)
        }
        frame 4 {
          w144 = "\n\n        ! dont stop inside the model\n        MoveL Offs(pStart,0,0,"  # ! dont stop inside the model         MoveL Offs(pStart,0,0,
          n168 = local read "SET_term_z_offs"() -> (w136:dbl)
          n169 = local read "SET_zone"() -> (w133:i32)
          n170 = Add(x=w136, y=w140) -> (x+y=w137:dbl)
          n171 = local read "SET_tool"() -> (w130:string)
          n172 = Number To Decimal String(number=w133) -> (decimal integer string=w131:string)  [unwired: 1 in]
          n173 = Number To Fractional String(use system decimal point (T)=FALSE ("Systemdezimalzeichen verwenden (T)"), number=w137, precision (6)=i16 3 ("Genauigkeit (6)")) -> (F-format string=w138:string)  [unwired: 1 in]
          n174 = Concatenate Strings(w144, w138, "),", w142, ",z", w131, "," ("String"), w130, ";" ("String")) -> (w145:string)
        }
      }
      n175 = local read "SET_tool"() -> (w63:string)
      n176 = Concatenate Strings(w43, "_0" ("string")) -> (w61:string)
      n177 = Concatenate Strings(w43, "_0.mod" ("string")) -> (w67:string)
      n178 = Build Path(base path=w42, name or relative path=w67) -> (appended path=w58:path)
      n179 = Strip Path(path=w42) -> (name=w41:string)  [unwired: 1 out]
      n180 = Concatenate Strings("MODULE " ("string"), w61, "\n    \n    LOCAL CONST robtarget pStart := [[7307.65,6245.57,-154.18],[0.625267,-0.348239,0.608726,0.342379],[1,0,-1,1],[6200.01,9E+09,9E+09,9E+09,9E+09,9E+09]];" ("string"), w37, "\n    \n    PROC ", w61, "_main()\n \n        ! move to pStart for teaching\n        MoveL pStart,v200,fine," ("string"), w63, ";\n\n        ! start printjob relative to pStart" ("string")) -> (w59:string)
      n181 = Increment(x=w39) -> (x+1=w40:i32)
      n182 = for {
        N: w40 -> [w188]
        shift-right: [w186] -> w57
        shift-left: w59 -> [w185]
        tunnel: w43 -> [w190]
        tunnel: w41 -> [w191]
        i -> [w187]
        n183 = Decrement(x=w188) -> (x-1=w181:i32)
        n184 = Not Equal To 0?(x=w187) -> (x != 0?=w192:bool)
        n185 = Greater?(x=w181, y=w187) -> (0:w189:bool)
        n186 = case shown="True" w189 {
          tunnel: w191 -> [_ w204]
          tunnel: w190 -> [_ w203]
          tunnel: w187 -> [_ w201]
          tunnel: ["" w197] -> w183
          tunnel: ["" w196] -> w184
          frame False {
          }
          frame True {
            w195 = "\r"
            n187 = Increment(x=w201) -> (x+1=w202:i32)
            n188 = Number To Decimal String(number=w202) -> (decimal integer string=w199:string)  [unwired: 1 in]
            n189 = Increment(x=w201) -> (x+1=w210:i32)
            n190 = Concatenate Strings("\n        WaitLoad load", w199, ";" ("string"), w195, w195) -> (w197:string)
            n191 = Concatenate Strings("\n        StartLoad \\Dynamic, \"HOME:/", w204, "/\" \\File:=\"" ("String"), w203) -> (w205:string)
            n192 = Number To Decimal String(number=w210) -> (decimal integer string=w209:string)  [unwired: 1 in]
            n193 = Concatenate Strings(w205, "_" ("string"), w209, ".mod\", load" ("string"), w209, ";") -> (w196:string)
          }
        }
        n194 = case shown="True" w192 {
          tunnel: w187 -> [_ w226]
          tunnel: w190 -> [_ w232]
          tunnel: w191 -> [_ w224]
          tunnel: w190 -> [_ w221]
          tunnel: w187 -> [_ w220]
          tunnel: ["" w215] -> w182
          frame False {
          }
          frame True {
            n195 = Number To Decimal String(number=w226) -> (decimal integer string=w230:string)  [unwired: 1 in]
            n196 = Number To Decimal String(number=w220) -> (decimal integer string=w219:string)  [unwired: 1 in]
            n197 = Concatenate Strings(w232, "_" ("string"), w230) -> (w228:string)
            n198 = Concatenate Strings(w221, "_" ("string"), w219) -> (w218:string)
            n199 = Concatenate Strings("\n        %\"", w228, ":", w228, "_main\"%(pStart);" ("String")) -> (w217:string)
            n200 = Concatenate Strings("\n        UnLoad \"HOME:/", w224, "/\" \\File:=\"" ("String"), w218, ".mod\";" ("string")) -> (w216:string)
            n201 = Concatenate Strings(w217, w216) -> (w215:string)
          }
        }
        n202 = Concatenate Strings(w185, w184, w182, w183) -> (w186:string)
      }
      n203 = while {
        tunnel: [w153] -> w48
        stop <- w153 stop-if-true
        n204 = local read "OUT_choice"() -> (w153:bool)
      }
      n205 = Concatenate Strings(w57, w33, "\n\n    STOP;\n        \n    ENDPROC\n    \nENDMODULE" ("string")) -> (w55:string)
      n206 = case shown="True" w48 {
        tunnel: w58 -> [_ w158]
        tunnel: w55 -> [_ w157]
        frame False {
        }
        frame True {
          n207 = Open/Create/Replace File(file path (use dialog)=w158, error in=errorcluster {"status"=FALSE, "code"=0, "source"=""}, operation (0:open)=T1."replace or create", access (0:read/write)=enum16{"read/write", "read-only", "write-only"}."read/write") -> (refnum out=w161:refnum<file>, error out=w162:errorcluster)  [unwired: 2 in, 1 out]
          n208 = Write to Text File(file (use dialog)=w161, text=w157, error in=w162) -> (refnum out=w163:refnum<file>, error out=w164:errorcluster)  [unwired: 1 in, 1 out]
          n209 = Close File(refnum=w163, error in=w164) -> ()  [unwired: 2 out]
        }
      }
      n210 = local write "OUT_rapid"(w55) -> ()
    }
    frame False {
      n211 = local read "SET_tool"() -> (w1116:string)
      n212 = local read "FILE_name_new"() -> (w1122:string)
      n213 = Empty String/Path?(string/path=w1122) -> (empty?=w1125:bool)
      n214 = case shown="True" w1125 {
        tunnel: w1126 -> [_ w1158]
        tunnel: w1122 -> [w1157 _]
        tunnel: [w1156 w1160] -> w1120
        tunnel: [w1157 w1158] -> w1124
        frame False {
          n215 = Concatenate Strings(w1157, ".mod" ("string")) -> (w1156:string)
        }
        frame True {
          n216 = Concatenate Strings(w1158, "_RAPID.mod" ("string")) -> (w1160:string)
        }
      }
      n217 = Concatenate Strings("MODULE ", w1124, "\n    \n    LOCAL CONST robtarget pStart := [[7307.65,6245.57,-154.18],[0.625267,-0.348239,0.608726,0.342379],[1,0,-1,1],[6200.01,9E+09,9E+09,9E+09,9E+09,9E+09]];\n    \n    PROC ", w1124, "_main()\n \n        ! move to pStart for teaching\n        MoveL pStart,v200,fine,", w1116, ";\n\n        ! start printjob relative to pStart" ("string")) -> (w1127:string)
      n218 = Empty String/Path?(string/path=w1123) -> (empty?=w1131:bool)
      n219 = case shown="False" w1131 {
        tunnel: w1123 -> [w1179 _]
        tunnel: w1127 -> [w1178 _]
        tunnel: [w1177 w2031] -> w1112
        tunnel: "       \n    ENDPROC\n    \nENDMODULE" -> [w1166 _]
        frame False {
          w1168 = 0.0
          n220 = while {
            shift-right: [w1347] -> _
            shift-left: w1179 -> [w1349]
            shift-right: [w1343] -> w1176
            shift-left: w1178 -> [w1344]
            tunnel: [w1339] -> w1175
            shift-right: [w1326] -> _
            shift-left: w1168 -> [w1324]
            shift-right: [w1325] -> _
            shift-left: w1168 -> [w1323]
            shift-right: [w1292] -> _
            shift-left: w1168 -> [w1290]
            shift-right: [w1253] -> _
            shift-left: "0" ("whole match") -> [w1316]
            shift-right: [w1254] -> _
            shift-left: "0" ("whole match") -> [w1303]
            shift-right: [w1248] -> _
            shift-left: "0" ("whole match") -> [w1302]
            shift-right: [w1282] -> _
            shift-left: "0" ("whole match") -> [w1301]
            shift-right: [w1273] -> _
            shift-left: "0" ("whole match") -> [w1300]
            shift-right: [w1277] -> _
            shift-left: 0.0 -> [w1275]
            shift-right: [w1269] -> _
            shift-left: 180.0 -> [w1270]
            tunnel: [w1250] -> w1162
            tunnel: [w1247] -> w1163
            stop <- w1339 stop-if-true
            w1258 = FALSE ("Systemdezimalzeichen verwenden (T)")
            w1256 = FALSE ("Systemdezimalzeichen verwenden (T)")
            w1274 = "0.0"
            w1296 = FALSE ("use system decimal point (T)")
            w1329 = ","
            n221 = local write "CONV_running"(TRUE ("running")) -> ()
            n222 = Match Pattern(string=w1349, regular expression="\n") -> (before substring=w1346:string, after substring=w1347:string)  [unwired: 1 in, 2 out]
            n223 = Match Pattern(string=w1346, regular expression="G1") -> (after substring=w1299:string)  [unwired: 1 in, 3 out]
            n224 = Empty String/Path?(string/path=w1299) -> (empty?=w1342:bool)
            n225 = xnode "Match Regular Expression"("input string"=w1299, "regular expression"="X-?\\d+.?[\\d+]?") -> ("whole match"=w1317:string)  [unwired: 4 in, 4 out]
            n226 = xnode "Match Regular Expression"("input string"=w1299, "regular expression"="Y-?\\d+.?[\\d+]?") -> ("whole match"=w1315:string)  [unwired: 4 in, 4 out]
            n227 = xnode "Match Regular Expression"("input string"=w1299, "regular expression"="Z-?\\d+.?[\\d+]?") -> ("whole match"=w1310:string)  [unwired: 4 in, 4 out]
            n228 = xnode "Match Regular Expression"("input string"=w1299, "regular expression"="E\\d+.?[\\d+]?") -> ("whole match"=w1309:string)  [unwired: 4 in, 4 out]
            n229 = xnode "Match Regular Expression"("input string"=w1299, "regular expression"="F\\d+.?[\\d+]?") -> ("whole match"=w1304:string)  [unwired: 4 in, 4 out]
            n230 = Empty String/Path?(string/path=w1317) -> (empty?=w1318:bool)
            n231 = Empty String/Path?(string/path=w1315) -> (empty?=w1314:bool)
            n232 = Empty String/Path?(string/path=w1310) -> (empty?=w1311:bool)
            n233 = Empty String/Path?(string/path=w1309) -> (empty?=w1308:bool)
            n234 = Empty String/Path?(string/path=w1304) -> (empty?=w1305:bool)
            n235 = local read "SET_movtype"() -> (w1268:u16)
            n236 = case shown="True" w1318 {
              tunnel: w1317 -> [w1899 _]
              tunnel: [w1897 w1900] -> w1253
              tunnel: w1316 -> [_ w1900]
              frame False {
                n237 = String Subset(string=w1899, offset (0)=1) -> (substring=w1897:string)  [unwired: 1 in]
              }
              frame True {
              }
            }
            n238 = Fract/Exp String To Number(use system decimal point (T)=w1296, string=w1253) -> (number=w1326:dbl)  [unwired: 2 in, 1 out]
            n239 = case shown="False" w1314 {
              tunnel: w1315 -> [w1778 _]
              tunnel: [w1776 w1779] -> w1254
              tunnel: w1303 -> [_ w1779]
              frame False {
                n240 = String Subset(string=w1778, offset (0)=1) -> (substring=w1776:string)  [unwired: 1 in]
              }
              frame True {
              }
            }
            n241 = Fract/Exp String To Number(use system decimal point (T)=w1296, string=w1254) -> (number=w1325:dbl)  [unwired: 2 in, 1 out]
            n242 = case shown="False" w1311 {
              tunnel: w1310 -> [w1657 _]
              tunnel: [w1655 w1658] -> w1248
              tunnel: w1302 -> [_ w1658]
              frame False {
                n243 = String Subset(string=w1657, offset (0)=1) -> (substring=w1655:string)  [unwired: 1 in]
              }
              frame True {
              }
            }
            n244 = Fract/Exp String To Number(use system decimal point (T)=w1296, string=w1248) -> (number=w1292:dbl)  [unwired: 2 in, 1 out]
            n245 = case shown="False" w1308 {
              tunnel: w1309 -> [w1536 _]
              tunnel: [w1534 w1537] -> w1282
              tunnel: w1301 -> [_ w1537]
              frame False {
                n246 = String Subset(string=w1536, offset (0)=1) -> (substring=w1534:string)  [unwired: 1 in]
              }
              frame True {
              }
            }
            n247 = Fract/Exp String To Number(use system decimal point (T)=FALSE, string=w1282) -> (number=w1276:dbl)  [unwired: 2 in, 1 out]
            n248 = case shown="True" w1305 {
              tunnel: w1304 -> [w1415 _]
              tunnel: [w1413 w1416] -> w1273
              tunnel: w1300 -> [_ w1416]
              frame False {
                n249 = String Subset(string=w1415, offset (0)=1) -> (substring=w1413:string)  [unwired: 1 in]
              }
              frame True {
              }
            }
            n250 = Fract/Exp String To Number(use system decimal point (T)=FALSE ("Systemdezimalzeichen verwenden (T)"), string=w1273) -> (number=w1298:dbl)  [unwired: 2 in, 1 out]
            n251 = Subtract(x=w1326, y=w1324) -> (x-y=w1321:dbl)
            n252 = Subtract(x=w1325, y=w1323) -> (x-y=w1322:dbl)
            n253 = Subtract(x=w1292, y=w1290) -> (x-y=w1291:dbl)
            n254 = Subtract(x=w1276, y=w1275) -> (x-y=w1278:dbl)
            n255 = Add(x=w1276, y=w1275) -> (x+y=w1277:dbl)
            n256 = Divide(x=w1298, y=10.0) -> (x/y=w1271:dbl)
            n257 = formula code="float X_ARC = 0;  float Z_ARC = 0;\n          float Rx = 0;  float Ry = 0;  float Rz = 0;\n        \n          if(  (VX == 0) && (VY == 0)  )   {\n                X_ARC = 0;\n                Z_ARC = 0;\n          }   else   {\n                X_ARC = acos(  VX / (  sqrt(  pow(VX,2) + pow(VY,2) ) ) );\n                Z_ARC = acos(  VZ / (  sqrt(  pow(VX,2) + pow(VY,2) + pow(VZ,2) ) ) );\n          }\n        \n          X_ARC = X_ARC * 180 / 3.141592653589;\n          if(VY < 0) X_ARC += 180;"("VX"=w1321, "VY"=w1322, "VZ"=w1291) -> ("X_ARC"=w1289:dbl, "Z_ARC"=w1287:dbl)
            n258 = Equal To 0?(x=w1271) -> (x = 0?=w1272:bool)
            n259 = Absolute Value(x=w1278) -> (abs(x)=w1246:dbl)
            n260 = case shown="False" w1272 {
              tunnel: w1271 -> [w1350 _]
              tunnel: [w1350 w1351] -> w1269
              tunnel: w1270 -> [_ w1351]
              frame False {
              }
              frame True {
              }
            }
            n261 = formula code="int16 v1 = F;\n   float v2 = 50.6 + 0.084 * F;\n   int16 v3 = F;\n   int16 v4 = 72 +  + 0.113 * F;\n   if(v4 > 180) v4 = 180;"("F"=w1269) -> ("v1"=w1338:i16, "v2"=w1337:dbl, "v3"=w1335:i16, "v4"=w1334:i16)
            n262 = case shown="0, Standard" w1268 {
              tunnel: ["        MoveL" "        MoveJ"] -> w1341
              frame 0, Default {
              }
              frame 1 {
              }
            }
            n263 = local read "SET_x_offs"() -> (w1262:dbl)
            n264 = local read "SET_y_offs"() -> (w1261:dbl)
            n265 = Number To Fractional String(number=w1246, precision (6)=i16 2) -> (F-format string=w1279:string)  [unwired: 2 in]
            n266 = Fract/Exp String To Number(use system decimal point (T)=w1256, string=w1253) -> (number=w1264:dbl)  [unwired: 2 in, 1 out]
            n267 = Fract/Exp String To Number(use system decimal point (T)=w1258, string=w1254) -> (number=w1259:dbl)  [unwired: 2 in, 1 out]
            n268 = local read "SET_tool_angl"() -> (w1266:bool)
            n269 = Add(x=w1264, y=w1262) -> (x+y=w1263:dbl)
            n270 = Add(x=w1259, y=w1261) -> (x+y=w1260:dbl)
            n271 = Number To Fractional String(number=w1289, precision (6)=i16 2) -> (F-format string=w1285:string)  [unwired: 2 in]
            n272 = Number To Fractional String(use system decimal point (T)=w1256, number=w1263, precision (6)=i16 3 ("Genauigkeit (6)")) -> (F-format string=w1252:string)  [unwired: 1 in]
            n273 = Number To Fractional String(use system decimal point (T)=w1258, number=w1260, precision (6)=i16 3 ("Genauigkeit (6)")) -> (F-format string=w1251:string)  [unwired: 1 in]
            n274 = Number To Fractional String(number=w1287, precision (6)=i16 2) -> (F-format string=w1286:string)  [unwired: 2 in]
            n275 = local read "SET_zone"() -> (w1265:i32)
            n276 = To Word Integer(number=w1337) -> (16bit integer=w1336:i16)
            n277 = case shown="0" w1265 {
              tunnel: ["z1" "z2" "z5" "z10" "z20" "z50" "z100" "z200" "z300" "z400" "z500"] -> w1340
              frame 0 {
              }
              frame 1, 2 {
              }
              frame 3..5 {
              }
              frame 6..10, Default {
              }
              frame 11..20 {
              }
              frame 21..50 {
              }
              frame 51..100 {
              }
              frame 101..200 {
              }
              frame 201..300 {
              }
              frame 301..400 {
              }
              frame 401..500 {
              }
            }
            n278 = Number To Decimal String(number=w1338) -> (decimal integer string=w1332:string)  [unwired: 1 in]
            n279 = Number To Decimal String(number=w1336) -> (decimal integer string=w1331:string)  [unwired: 1 in]
            n280 = Number To Decimal String(number=w1335) -> (decimal integer string=w1330:string)  [unwired: 1 in]
            n281 = Number To Decimal String(number=w1334) -> (decimal integer string=w1328:string)  [unwired: 1 in]
            n282 = Concatenate Strings("     !Z_ARC: ", w1286, "°      X_ARC: ", w1285, "°      EL: " ("string"), w1279, "mm" ("string")) -> (w1283:string)
            n283 = Concatenate Strings("[", w1332, w1329, w1331, w1329, w1330, w1329, w1328, "]") -> (w1250:string)
            n284 = case shown="False" w1266 {
              tunnel: w1344 -> [w1361 w1390]
              tunnel: [w1360 w1389] -> w1343
              tunnel: w1342 -> [w1359 w1388]
              tunnel: w1341 -> [w1358 w1387]
              tunnel: w1340 -> [w1357 w1386]
              tunnel: w1250 -> [w1356 w1385]
              tunnel: w1251 -> [w1355 w1384]
              tunnel: w1252 -> [w1354 w1383]
              tunnel: w1248 -> [w1353 w1382]
              tunnel: w1283 -> [w1352 w1381]
              tunnel: w1274 -> [_ w1380]
              tunnel: w1274 -> [_ w1379]
              tunnel: w1274 -> [_ w1378]
              frame False {
                n285 = case shown="False" w1359 {
                  tunnel: w1361 -> [w1376 w1377]
                  tunnel: w1354 -> [w1373 _]
                  tunnel: w1355 -> [w1372 _]
                  tunnel: w1353 -> [w1371 _]
                  tunnel: w1356 -> [w1370 _]
                  tunnel: [w1369 w1377] -> w1360
                  tunnel: w1358 -> [w1367 _]
                  tunnel: w1357 -> [w1365 _]
                  tunnel: w1352 -> [w1362 _]
                  frame False {
                    w1364 = ","
                    n286 = local read "SET_tool"() -> (w1363:string)
                    n287 = Concatenate Strings(w1376, "\r", w1367, " Offs(pStart,", w1373, w1364, w1372, w1364, w1371, ")" ("string"), w1364, w1370, w1364, w1365, w1364, w1363, ";" ("string"), w1362) -> (w1369:string)
                  }
                  frame True {
                  }
                }
              }
              frame True {
                n288 = case shown="False" w1388 {
                  tunnel: w1390 -> [w1411 w1412]
                  tunnel: w1383 -> [w1408 _]
                  tunnel: w1384 -> [w1407 _]
                  tunnel: w1382 -> [w1406 _]
                  tunnel: w1385 -> [w1405 _]
                  tunnel: [w1404 w1412] -> w1389
                  tunnel: w1387 -> [w1402 _]
                  tunnel: w1386 -> [w1400 _]
                  tunnel: w1381 -> [w1397 _]
                  tunnel: w1380 -> [w1396 _]
                  tunnel: w1379 -> [w1395 _]
                  tunnel: w1378 -> [w1394 _]
                  frame False {
                    w1399 = ","
                    n289 = local read "SET_tool"() -> (w1398:string)
                    n290 = Concatenate Strings(w1411, "\r", w1402, " RelTool(pStart,", w1408, w1399, w1407, w1399, w1406, "\\Rx:=" ("string"), w1396, "\\Ry:=" ("string"), w1395, "\\Rz:=" ("string"), w1394, ")" ("string"), w1399, w1405, w1399, w1400, w1399, w1398, ";" ("string"), w1397) -> (w1404:string)
                  }
                  frame True {
                  }
                }
              }
            }
            n291 = Empty String/Path?(string/path=w1349) -> (empty?=w1339:bool)
            n292 = Fract/Exp String To Number(use system decimal point (T)=FALSE ("Systemdezimalzeichen verwenden (T)"), string=w1248) -> (number=w1247:dbl)  [unwired: 2 in, 1 out]
          }
          n293 = Not(x=w1175) -> (.not. x?=w1174:bool)
          n294 = local write "CONV_running"(w1174) -> ()
          n295 = local read "SET_term_moc"() -> (w1164:u16)
          n296 = case shown="1" w1164 {
            tunnel: ["" w1196 w1212 w1228 w1244] -> w1161
            tunnel: w1162 -> [_ w1193 w1209 w1225 w1241]
            tunnel: w1163 -> [_ w1191 w1207 w1223 w1239]
            frame 0, Default {
            }
            frame 1 {
              w1195 = "\n\n        ! dont stop inside the model\n        MoveL Offs(pStart,50.0,50.0,"  # ! dont stop inside the model         MoveL Offs(pStart,50.0,50.0,
              n297 = local read "SET_term_z_offs"() -> (w1187:dbl)
              n298 = local read "SET_zone"() -> (w1184:i32)
              n299 = Add(x=w1187, y=w1191) -> (x+y=w1188:dbl)
              n300 = local read "SET_tool"() -> (w1182:string)
              n301 = Number To Decimal String(number=w1184) -> (decimal integer string=w1183:string)  [unwired: 1 in]
              n302 = Number To Fractional String(use system decimal point (T)=FALSE ("Systemdezimalzeichen verwenden (T)"), number=w1188, precision (6)=i16 3 ("Genauigkeit (6)")) -> (F-format string=w1189:string)  [unwired: 1 in]
              n303 = Concatenate Strings(w1195, w1189, "),", w1193, ",z", w1183, "," ("String"), w1182, ";" ("String")) -> (w1196:string)
            }
            frame 2 {
              w1211 = "\n\n        ! dont stop inside the model\n        MoveL Offs(pStart,-50.0,0.0,"  # ! dont stop inside the model         MoveL Offs(pStart,-50.0,0.0,
              n304 = local read "SET_term_z_offs"() -> (w1203:dbl)
              n305 = local read "SET_zone"() -> (w1200:i32)
              n306 = Add(x=w1203, y=w1207) -> (x+y=w1204:dbl)
              n307 = local read "SET_tool"() -> (w1197:string)
              n308 = Number To Decimal String(number=w1200) -> (decimal integer string=w1198:string)  [unwired: 1 in]
              n309 = Number To Fractional String(use system decimal point (T)=FALSE ("Systemdezimalzeichen verwenden (T)"), number=w1204, precision (6)=i16 3 ("Genauigkeit (6)")) -> (F-format string=w1205:string)  [unwired: 1 in]
              n310 = Concatenate Strings(w1211, w1205, "),", w1209, ",z", w1198, "," ("String"), w1197, ";" ("String")) -> (w1212:string)
            }
            frame 3 {
              w1227 = "\n\n        ! dont stop inside the model\n        MoveL Offs(pStart,0,-50.0,"  # ! dont stop inside the model         MoveL Offs(pStart,0,-50.0,
              n311 = local read "SET_term_z_offs"() -> (w1219:dbl)
              n312 = local read "SET_zone"() -> (w1216:i32)
              n313 = Add(x=w1219, y=w1223) -> (x+y=w1220:dbl)
              n314 = local read "SET_tool"() -> (w1213:string)
              n315 = Number To Decimal String(number=w1216) -> (decimal integer string=w1214:string)  [unwired: 1 in]
              n316 = Number To Fractional String(use system decimal point (T)=FALSE ("Systemdezimalzeichen verwenden (T)"), number=w1220, precision (6)=i16 3 ("Genauigkeit (6)")) -> (F-format string=w1221:string)  [unwired: 1 in]
              n317 = Concatenate Strings(w1227, w1221, "),", w1225, ",z", w1214, "," ("String"), w1213, ";" ("String")) -> (w1228:string)
            }
            frame 4 {
              w1243 = "\n\n        ! dont stop inside the model\n        MoveL Offs(pStart,0,0,"  # ! dont stop inside the model         MoveL Offs(pStart,0,0,
              n318 = local read "SET_term_z_offs"() -> (w1235:dbl)
              n319 = local read "SET_zone"() -> (w1232:i32)
              n320 = Add(x=w1235, y=w1239) -> (x+y=w1236:dbl)
              n321 = local read "SET_tool"() -> (w1229:string)
              n322 = Number To Decimal String(number=w1232) -> (decimal integer string=w1230:string)  [unwired: 1 in]
              n323 = Number To Fractional String(use system decimal point (T)=FALSE ("Systemdezimalzeichen verwenden (T)"), number=w1236, precision (6)=i16 3 ("Genauigkeit (6)")) -> (F-format string=w1237:string)  [unwired: 1 in]
              n324 = Concatenate Strings(w1243, w1237, "),", w1241, ",z", w1230, "," ("String"), w1229, ";" ("String")) -> (w1244:string)
            }
          }
          n325 = Concatenate Strings(w1176, w1161, w1166) -> (w1177:string)
        }
        frame True {
          w2031 = "File is empty!" ("message")
          n326 = One Button Dialog(message=w2031, button name ("OK")="End program") -> ()  [unwired: 1 out]
        }
      }
      n327 = Build Path(base path=w1121, name or relative path=w1120) -> (appended path=w1113:path)
      n328 = Open/Create/Replace File(file path (use dialog)=w1113, error in=errorcluster {"status"=FALSE, "code"=0, "source"=""}, operation (0:open)=T1."create", access (0:read/write)=enum16{"read/write", "read-only", "write-only"}."read/write") -> (refnum out=w1110:refnum<file>, error out=w1111:errorcluster)  [unwired: 2 in, 1 out]
      n329 = Unbundle(w1111) -> ("status"=w1114:bool)  [unwired: 2 out]
      n330 = case shown="True" w1114 {
        tunnel: w1113 -> [_ w1139]
        tunnel: w1112 -> [w1133 w1138]
        tunnel: w1111 -> [w1134 _]
        tunnel: w1110 -> [w1132 _]
        frame False {
          n331 = Write to Text File(file (use dialog)=w1132, text=w1133, error in=w1134) -> (refnum out=w1135:refnum<file>, error out=w1136:errorcluster)  [unwired: 1 in, 1 out]
          n332 = local write "OUT_rapid"(w1133) -> ()
          n333 = Close File(refnum=w1135, error in=w1136) -> (error out=w1137:errorcluster)  [unwired: 1 out]
          n334 = local write "ERR_write_file"(w1137) -> ()
        }
        frame True {
          n335 = flat-sequence {
            tunnel: w1139 -> [w1148]
            tunnel: w1138 -> [w1149]
            frame #0 {
              n336 = Two Button Dialog(message="CAUTION!\n\nFile with the same name\nalready exists. Do you want to\noverwrite?", 1:"EXIT PROGRAM" ("F button name (\"Cancel\")"), 2:"OVERWRITE" ("T button name (\"OK\")")) -> (T button?=w1140:bool)
              n337 = Not(x=w1140) -> (.not. x?=w1141:bool)
              n338 = Stop(stop? (T)=w1141) -> ()
            }
            frame #1 {
              n339 = Open/Create/Replace File(file path (use dialog)=w1148, error in=errorcluster {"status"=FALSE, "code"=0, "source"=""}, operation (0:open)=T1."replace or create", access (0:read/write)=enum16{"read/write", "read-only", "write-only"}."read/write") -> (refnum out=w1147:refnum<file>, error out=w1146:errorcluster)  [unwired: 2 in, 1 out]
              n340 = Write to Text File(file (use dialog)=w1147, text=w1149, error in=w1146) -> (refnum out=w1150:refnum<file>, error out=w1151:errorcluster)  [unwired: 1 in, 1 out]
              n341 = local write "OUT_rapid"(w1149) -> ()
              n342 = Close File(refnum=w1150, error in=w1151) -> (error out=w1152:errorcluster)  [unwired: 1 out]
              n343 = local write "ERR_write_file"(w1152) -> ()
            }
          }
        }
      }
    }
  }
